vi "dfd_Multirate Filter Param Validation.vi"(6 "raised cos?":bool, 7 "multirate factor":i32=4, 8 "error in (no error)":errorcluster, 9 "A Stop [dB]":dbl=80.0 format="%.2f", 10 "roll off":dbl=0.2 format="%.2f", 11 "order":i32=20) -> (0 "error out":errorcluster, 1 "dup A Stop [dB]":dbl=80.0 format="%.2f", 2 "dup roll off":dbl format="%.2f", 3 "dup order":i32=20)   [LabVIEW 2017, in "NI_DigFilter_Process.lvlib"]
uses:
  <vilib>/addons/Digital Filter Design/NI_DigFilter_Process.lvlib
  <vilib>/addons/Digital Filter Design/_Misc.llb/dfd_Error Handlers (Multiple).vi
  <vilib>/addons/Digital Filter Design/NI_DigFilterLicensed.lvlib
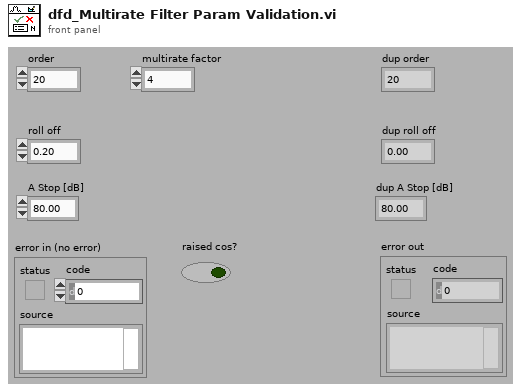
[diagram p1: front panel]
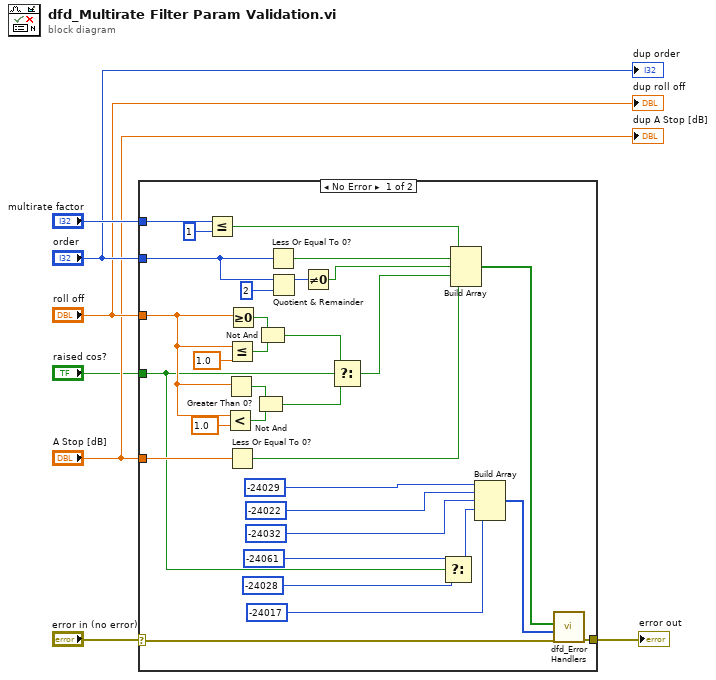
[diagram p0: block diagram]
diagram:
  n1 = case shown="No Error" "error in (no error)" {
    selector: "error in (no error)" -> [w29 w40]
    tunnel: "roll off" -> [w17 _]
    tunnel: "multirate factor" -> [w30 _]
    tunnel: [w39 w40] -> w6
    tunnel: "A Stop [dB]" -> [w26 _]
    tunnel: "order" -> [w21 _]
    tunnel: "raised cos?" -> [w11 _]
    frame No Error {
      n2 = Less Or Equal?(x=w30, y=1) -> (x <= y?=w34:bool)
      n3 = Less?(x=w17, y=1.0) -> (x < y?=w20:bool)
      n4 = Greater Than 0?(x=w17) -> (x > 0?=w19:bool)
      n5 = Less Or Equal?(x=w17, y=1.0) -> (x <= y?=w36:bool)
      n6 = Less Or Equal To 0?(x=w26) -> (x <= 0?=w28:bool)
      n7 = Greater Or Equal To 0?(x=w17) -> (x >= 0?=w37:bool)
      n8 = Not And(1:w20, 2:w19) -> (0:w15:bool)
      n9 = Not And(1:w36, 2:w37) -> (0:w16:bool)
      n10 = Less Or Equal To 0?(x=w21) -> (x <= 0?=w23:bool)
      n11 = Quotient & Remainder(x=w21, y=2) -> (x-y*floor(x/y)=w24:i32)  [unwired: 1 out]
      n12 = Not Equal To 0?(x=w24) -> (x != 0?=w22:bool)
      n13 = Select(t=w16, s=w11, f=w15) -> (s? t:f=w14:bool)
      n14 = Select(t=-24061 ("ERR_RCOS_ROLLOFF_RANGE"), s=w11, f=-24028 ("ERR_ROLLOFF_RANGE_WRONG")) -> (s? t:f=w8:i32)
      n15 = Build Array(w34, w23, w22, w14, w28) -> (w31:bool[])
      n16 = Build Array(-24029 ("ERR_#BAND_LE_ONE"), -24022 ("ERR_ORDER_LE_ZERO"), -24032 ("ERR_ORDER_ODD"), w8, -24017 ("ERR_dB_LE_ZERO")) -> (w32:i32[])
      n17 = call-poly <vilib>:"dfd_Error Handlers.vi"("error in (no error)"=w29, "error sources"=w32, "condition failed?"=w31) -> ("error out"=w39:errorcluster)  [unwired: 8 out]
    }
    frame Error {
    }
  }
  "error out" <- w6
  "dup roll off" <- "roll off"
  "dup order" <- "order"
  "dup A Stop [dB]" <- "A Stop [dB]"
